vi "Disconnect All.vi"(8 "error in (no error)":errorcluster, 11 "PIPXI40 Switching in":refnum<class "PIPX40 Relay.lvclass">) -> (0 "error out":errorcluster, 3 "PIPXI40 Switching out":refnum<class "PIPX40 Relay.lvclass">)   [LabVIEW 2020, in "Pickering.lvlib" / "PIPX40 Relay.lvclass"]
uses:
  PIPX40 Relay.lvclass
  D:/WSGitHub/RTFWK/Realization/PIPX40 Base/PIPX40 Base.lvclass
  PIPX40 Relay.lvclass/PIPX40 Relay.ctl
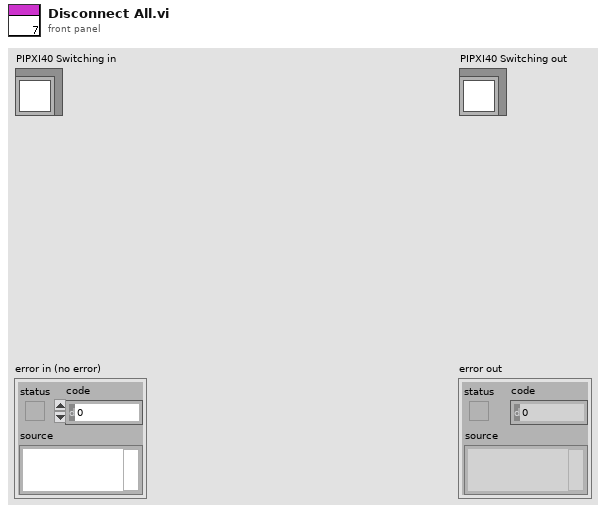
[diagram p1: front panel]
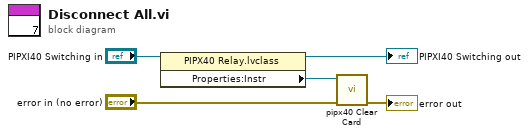
[diagram p0: block diagram]
diagram:
  n1 = property class="PIPX40 Relay.lvclass"(reference="PIPXI40 Switching in") -> (reference out=→"PIPXI40 Switching out":refnum<class "PIPX40 Relay.lvclass">, "Properties:Instr"=w2:refnum<visa-resource-name>)  [unwired: 1 in, 1 out]
  n2 = call <instrlib>:"pipx40 Clear Card.vi"("error in (no error)"="error in (no error)", "instrument handle"=w2) -> ("error out"=→"error out":errorcluster)  [unwired: 8 in, 1 out]
